vi "Update Display.vi"(6 "Priority Message? (F)":bool, 8 "error in":errorcluster, 11 "Message string":string) -> (0 "error out":errorcluster)   [LabVIEW 2014]
uses:
  Message Queue/Message Queue.lvlib
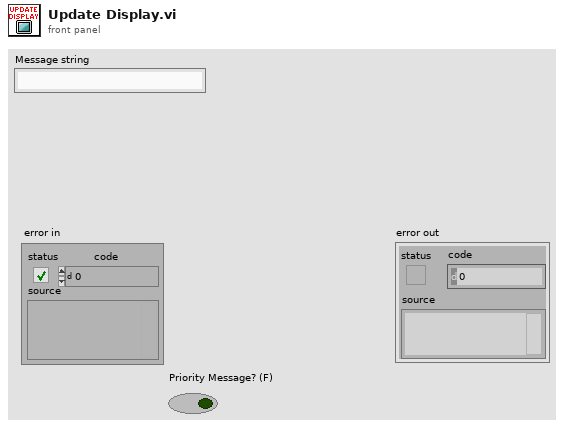
[diagram p1: front panel]
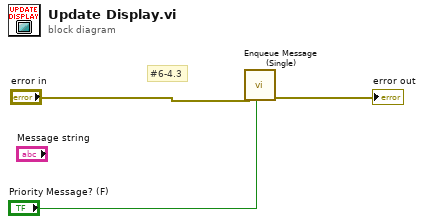
[diagram p0: block diagram]
diagram:
  # "#6-4.3"
  n1 = call "Enqueue Message (Single).vi"("Priority Message? (F)"="Priority Message? (F)", "error in (no error)"="error in") -> ("error out"=→"error out":errorcluster)  [unwired: 8 in, 1 out]
